vi "Untitled 1.vi"() -> ()   [LabVIEW 2011]
panel:
  in  "index":i32
  in  "Target Info":T1(array[cluster])
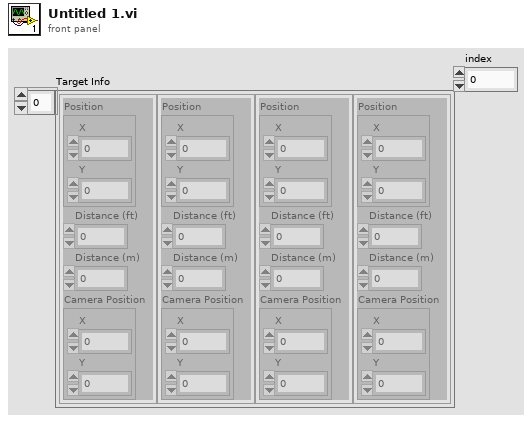
[diagram p1: front panel]
types:
  T1 = cluster{"Position":cluster{"X":dbl, "Y":dbl}, "Distance (ft)":dbl, "Distance (m)":dbl, "Camera Position":cluster{"X":dbl, "Y":dbl}}[]
  T2 = cluster{"Position":cluster{"X":dbl, "Y":dbl}, "Distance (ft)":dbl, "Distance (m)":dbl, "Camera Position":cluster{"X":dbl, "Y":dbl}}
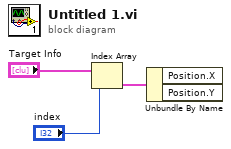
[diagram p0: block diagram]
diagram:
  n1 = Index Array(array="Target Info", index="index") -> (element=w1:T2)
  n2 = Unbundle By Name(w1) -> ()  [unwired: 2 out]
